vi "08_2.vi"() -> ()   [LabVIEW 2018]
uses:
  <userlib>/_OpenG.lib/array/array.llb/Remove Duplicates from 1D Array (I32)__ogtk.vi
panel:
  out "Solution":i32
  in  "Input":string
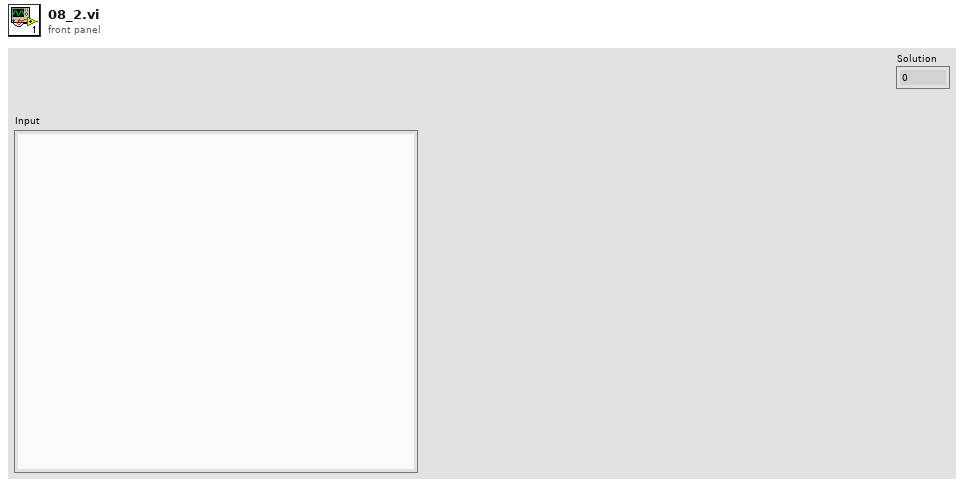
[diagram p1: front panel]
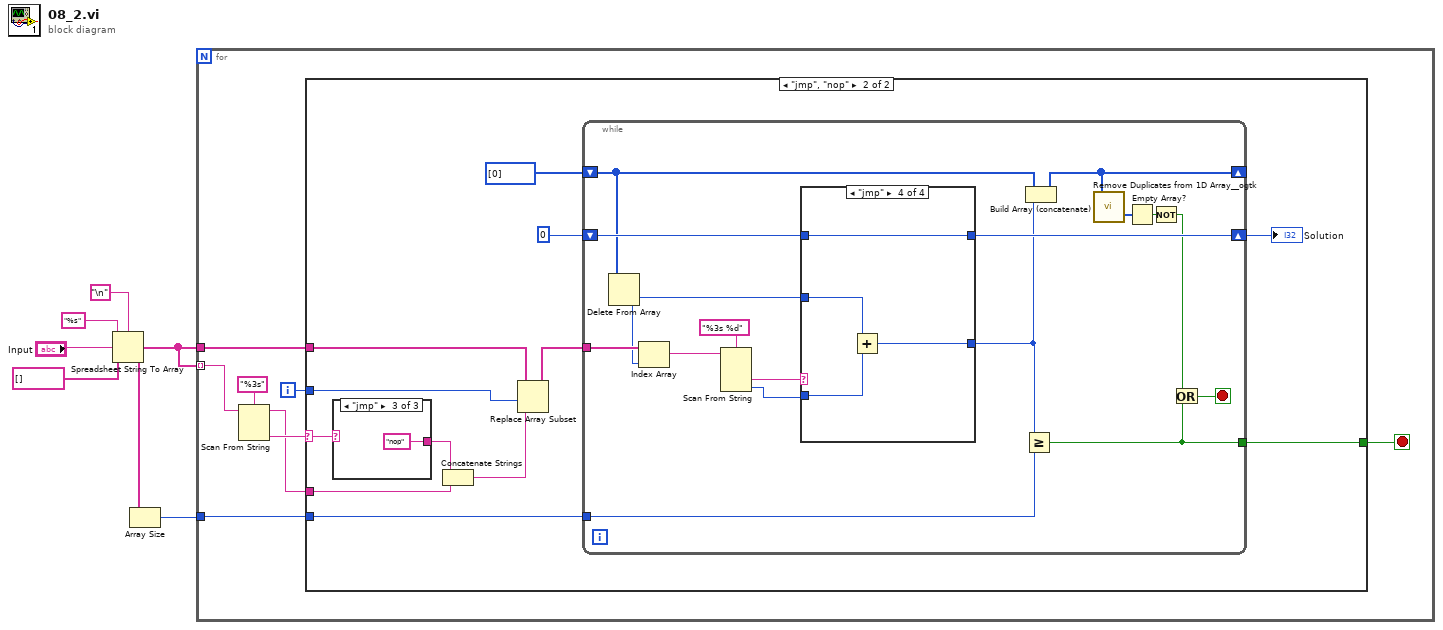
[diagram p0: block diagram]
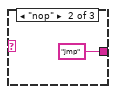
[diagram p4: hidden frame]
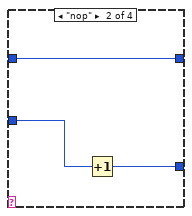
[diagram p6: hidden frame]
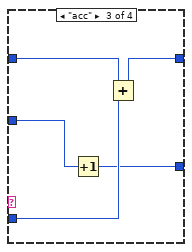
[diagram p7: hidden frame]
diagram:
  n1 = Spreadsheet String To Array(delimiter (Tab)="\n", format string="%s", spreadsheet string="Input", array type (2D Dbl)=string[] []) -> (array=w1:string[])
  n2 = Array Size(array=w1) -> (size(s)=w2:i32)
  n3 = for {
    tunnel: w1 -> [w14]
    tunnel: w2 -> [w13]
    tunnel: w1 -> [w11] mode=indexing
    i -> [w8]
    stop <- w7 stop-if-true
    n4 = Scan From String(format string="%3s", input string=w11) -> (remaining string=w9:string, output 1=w10:string)  [unwired: 3 in, 2 out]
    n5 = case shown="\"jmp\", \"nop\"" w10 {
      selector: w10 -> [_ w22]
      tunnel: w14 -> [_ w18]
      tunnel: w13 -> [_ w23]
      tunnel: w9 -> [_ w20]
      tunnel: w8 -> [_ w16]
      tunnel: [_ w15] -> w7
      frame "acc", Default {
      }
      frame "jmp", "nop" {
        n6 = case shown="\"jmp\"" w22 {
          tunnel: [_ "jmp" "nop"] -> w21
          frame Default {
          }
          frame "nop" {
          }
          frame "jmp" {
          }
        }
        n7 = Concatenate Strings(w21, w20) -> (w17:string)
        n8 = Replace Array Subset(array=w18, new element=w17, index=w16) -> (w19:string[])
        n9 = while {
          tunnel: w19 -> [w44]
          shift-right: [w40] -> w24
          shift-left: 0 -> [w41]
          shift-right: [w36] -> _
          shift-left: i32[] [0] -> [w35]
          tunnel: w23 -> [w33]
          tunnel: [w29] -> w15
          stop <- w31 stop-if-true
          n10 = Delete From Array(array=w35) -> (deleted portion=w39:i32)  [unwired: 2 in, 1 out]
          n11 = Index Array(array=w44, index=w39) -> (element=w43:string)
          n12 = Scan From String(format string="%3s %d", input string=w43) -> (output 1=w42:string, output 2=w37:i32)  [unwired: 4 in, 3 out]
          n13 = case shown="\"jmp\"" w42 {
            tunnel: w41 -> [w47 w50 w53 w59]
            tunnel: [w47 w50 w51 w59] -> w40
            tunnel: w39 -> [w46 w49 w55 w57]
            tunnel: w37 -> [_ _ w54 w58]
            tunnel: [w46 w48 w52 w56] -> w34
            frame Default {
            }
            frame "nop" {
              n14 = Increment(x=w49) -> (x+1=w48:i32)
            }
            frame "acc" {
              n15 = Increment(x=w55) -> (x+1=w52:i32)
              n16 = Add(x=w53, y=w54) -> (x+y=w51:i32)
            }
            frame "jmp" {
              n17 = Add(x=w57, y=w58) -> (x+y=w56:i32)
            }
          }
          n18 = Greater Or Equal?(x=w34, y=w33) -> (x >= y?=w29:bool)
          n19 = Build Array (concatenate)(w35, w34) -> (w36:i32[])
          n20 = call-poly <userlib>:"Remove Duplicates from 1D Array__ogtk.vi"("Input Array"=w36) -> ("indices of removed elements"=w38:i32[])  [unwired: 1 out]
          n21 = Empty Array?(array=w38) -> (empty?=w32:bool)
          n22 = Not(x=w32) -> (.not. x?=w30:bool)
          n23 = Or(x=w30, y=w29) -> (x .or. y?=w31:bool)
        }
        "Solution" <- w24
      }
    }
  }
